vi "Configure Voltage.vi"(8 "error in (no error)":errorcluster, 10 "Set Voltage":dbl format="%.1g", 11 "VISA resource name":refnum<visa-resource-name>) -> (0 "error out":errorcluster, 3 "VISA resource name out":refnum<visa-resource-name>)   [LabVIEW 2021, in "BK Precision 169XB.lvlib"]
doc: "Configures over current protection (OCP). Specify the output current limit value and the behavior of the power supply when the output current is greater than or equal to that value."
uses:
  BK Precision 169XB.lvlib
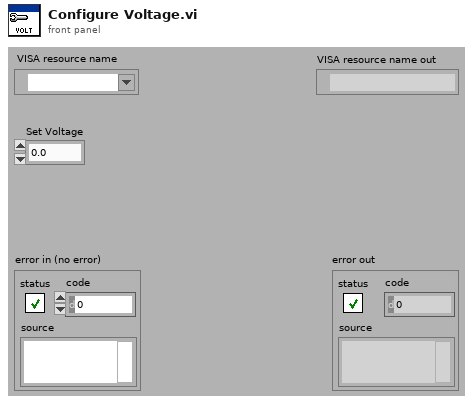
[diagram p1: front panel]
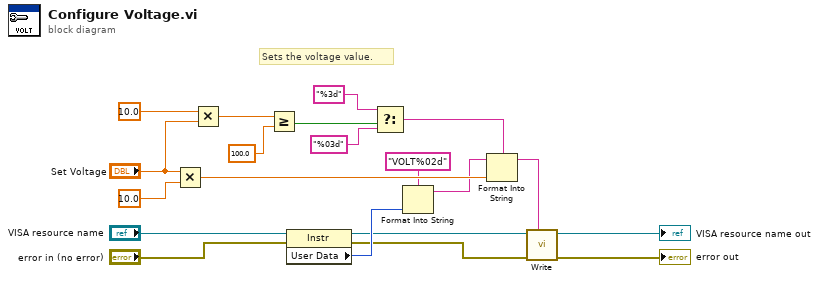
[diagram p0: block diagram]
diagram:
  # "Sets the voltage value."
  n1 = Multiply(x="Set Voltage", y=10.0) -> (x*y=w19:dbl)
  n2 = Multiply(x="Set Voltage", y=10.0) -> (x*y=w17:dbl)
  n3 = Greater Or Equal?(x=w17, y=100.0) -> (x >= y?=w15:bool)
  n4 = property class="Instr"(reference="VISA resource name", error in="error in (no error)") -> (reference out=w3:refnum<visa-resource-name>, error out=w2:errorcluster, "User Data"=w6:u32)
  n5 = Select(t="%3d" ("format string"), s=w15, f="%03d" ("format string")) -> (s? t:f=w12:string)
  n6 = Format Into String(format string="VOLT%02d", w6) -> (resulting string=w1:string)  [unwired: 2 in, 1 out]
  n7 = Format Into String(format string=w12, initial string=w1, w19) -> (resulting string=w10:string)  [unwired: 1 in, 1 out]
  n8 = call "Write.vi"("Input String"=w10, "error in (no error)"=w2, "VISA resource name"=w3) -> ("error out"=→"error out":errorcluster, "VISA resource name out"=→"VISA resource name out":refnum<visa-resource-name>)  [unwired: 6 in, 1 out]
